vi "xiLIB - LoadPRMValue.vi"(6 "INI Refnum":T2, 7 "xiCam In":refnum<k24>, 8 "error in (no error)":errorcluster, 9 "key":string, 10 "section":string, 11 "PRM":T3) -> (0 "error out":errorcluster, 3 "Load_Result":T1, 4 "INI Refnum out":T2)   [LabVIEW 2015]
uses:
  <vilib>/Utility/config.llb/NI_LVConfig.lvlib
  <vilib>/Utility/config.llb/Read Key (Double).vi
  <vilib>/Utility/config.llb/Read Key (I32).vi
  Typedefs/xiLIB - PRM_Load_Result.ctl
  C:/GIT/Cameras3.x/Integrations/Labview/xiLib/xiLIB_32bit/xiLIB/xiCamLib/API/x86/xiApi.NET.dll
  xiLIB_32bit/xiLIB/xiCamLib/API/x86/xiApi.NET.dll
  <vilib>/Utility/config.llb/Config Data RefNum.ctl
  xiCam/PRM/PRM/PRM_v2.ctl
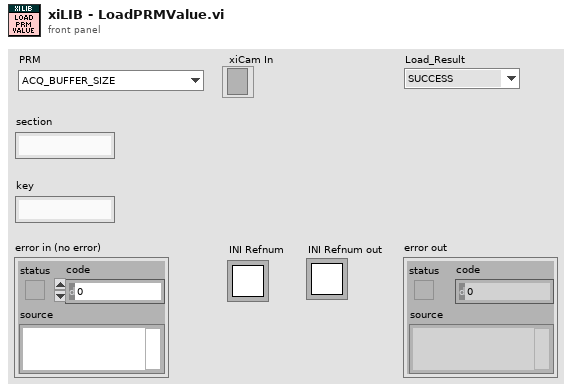
[diagram p1: front panel]
types:
  T1 = typedef "xiLIB - PRM_Load_Result.ctl" = enum16{"SUCCESS", "ERROR", "WARNING - Not Valid Parameter", "WARNING - Get Parameter"}
  T2 = typedef "NI_LVConfig.lvlib/Config Data RefNum.ctl" = refnum<k1>
  T3 = typedef "PRM_v2.ctl" = enum16{"ACQ_BUFFER_SIZE", "ACQ_FRAME_BURST_COUNT", "ACQ_TIMING_MODE", "ACQ_TRANSPORT_BUFFER_SIZE", "AE_MAX_LIMIT", "AEAG", "AEAG_LEVEL", "API_VERSION", "AG_MAX_LIMIT", "APPLY_CMS", "AUTO_BANDWIDTH_CALCULATION", "AUTO_WB", "AVAILABLE_BANDWIDTH", "AVAILABLE_BANDWIDTH_MAX", "AVAILABLE_BANDWIDTH_MIN", "BPC", "BUFFER_POLICY", "BUFFERS_QUEUE_SIZE", "CC_MATRIX_00", "CC_MATRIX_01", "CC_MATRIX_02", "CC_MATRIX_03", "CC_MATRIX_10", "CC_MATRIX_11", "CC_MATRIX_12", "CC_MATRIX_13", "CC_MATRIX_20", "CC_MATRIX_21", "CC_MATRIX_22", "CC_MATRIX_23", "CC_MATRIX_30", "CC_MATRIX_31", "CC_MATRIX_32", "CC_MATRIX_33", "CHIP_TEMP", "CMS", "COLOR_FILTER_ARRAY", "COOLING", "DEBOUNCE_EN", "DEBOUNCE_POL", "DEBOUNCE_T0", "DEBOUNCE_T1", "DEBUG_LEVEL", "DEFAULT_CC_MATRIX", "DEVICE_INSTANCE_PATH", "DEVICE_MODEL_ID", "DEVICE_NAME", "DEVICE_SN", "DEVICE_TYPE", "DEVICE_USER_ID", "DOWNSAMPLING", "DOWNSAMPLING_MAX", "DOWNSAMPLING_MIN", "DOWNSAMPLING_TYPE", "DRV_VERSION", "EXP_PRIORITY", "EXPOSURE", "EXPOSURE_DIRECT_UPDATE", "EXPOSURE_MAX", "EXPOSURE_MIN", "FFS_FILE_NAME", "FPGA1_VERSION", "FRAMERATE", "FRAMERATE_MAX", "FRAMERATE_MIN", "FREE_FFS_SIZE", "GAIN", "GAIN_DIRECT_UPDATE", "GAIN_MAX", "GAIN_MIN", "GAMMAC", "GAMMAY", "GPI_LEVEL", "GPI_MODE", "GPI_SELECTOR", "GPI_SELECTOR_MAX", "GPI_SELECTOR_MIN", "GPO_MODE", "GPO_SELECTOR", "GPO_SELECTOR_MAX", "GPO_SELECTOR_MIN", "HDR", "HDR_T1", "HDR_T2", "HEIGHT", "HEIGHT_MAX", "HEIGHT_MIN", "HOUSE_TEMP", "IMAGE_DATA_FORMAT", "IMAGE_IS_COLOR", "INPUT_CMS_PROFILE", "IS_COOLED", "IS_DEVICE_EXIST", "KNEEPOINT1", "KNEEPOINT2", "LED_MODE", "LED_SELECTOR", "LED_SELECTOR_MAX", "LED_SELECTOR_MIN", "LIMIT_BANDWIDTH", "LIMIT_BANDWIDTH_MAX", "LIMIT_BANDWIDTH_MIN", "LUT_EN", "LUT_INDEX", "LUT_INDEX_MAX", "LUT_INDEX_MIN", "LUT_VALUE", "LUT_VALUE_MAX", "LUT_VALUE_MIN", "MANUAL_WB", "MCU1_VERSION", "MCU2_VERSION", "OFFSET_X", "OFFSET_X_MAX", "OFFSET_X_MIN", "OFFSET_Y", "OFFSET_Y_MAX", "OFFSET_Y_MIN", "OUTPUT_CMS_PROFILE", "OUTPUT_DATA_BIT_DEPTH", "OUTPUT_DATA_PACKING", "READ_FILE_FFS", "RECENT_FRAME", "SENSOR_DATA_BIT_DEPTH", "SENSOR_MODE", "SENSOR_TAPS", "SHARPNESS", "SHUTTER_TYPE", "TARGET_TEMP", "TRG_DELAY", "TRG_SELECTOR", "TRG_SOFTWARE", "TRG_SOURCE", "USED_FFS_SIZE", "WB_KB", "WB_KG", "WB_KR", "WIDTH", "WIDTH_MAX", "WIDTH_MIN", "WRITE_FILE_FFS", "ACQ_BUFFER_SIZE_UNIT", "ACQ_TRANSPORT_BUFFER_COMMIT", "AEAG_ROI_HEIGHT", "AEAG_ROI_OFFSET_X", "AEAG_ROU_OFFSET_Y", "AEAG_ROI_WIDTH", "API_CONTEXT_LIST", "BINNING_HORIZONTAL", "BINNING_SELECTOR", "BINNING_VERTICAL", "COLUMN_FPN_CORRECTION", "COUNTER_SELECTOR", "COUNTER_VALUE", "DECIMATION_HORIZONTAL", "DECIMATION_SELECTOR", "DECIMATION_VERTICAL", "DEVICE_ID", "DEVICE_LOCATION_PATH", "DEVICE_MANIFEST", "DEVICE_RESET", "DEVICE_SENS_SN", "EXPOSURE_BURST_COUNT", "FFS_ACCESS_KEY", "GAIN_SELECTOR", "HW_REVISION", "IMAGE_BLACK_LEVEL", "IMAGE_DATA_BIT_DEPTH", "IMAGE_DATA_FORMAT_RGB32_ALPHA", "IMAGE_PAYLOAD_SIZE", "LENS_APERTURE_VALUE", "LENS_FEATURE", "LENS_FEATURE_SELECTOR", "LENS_FOCAL_LENGTH", "LENS_FOCUS_DISTANCE", "LENS_FOCUS_MOVE", "LENS_FOCUS_MOVEMENT_VALUE", "LENS_MODE", "OUTPUT_DATA_PACKING_TYPE", "SENSOR_CLOCK_FREQ_HZ", "SENSOR_CLOCK_FREQ_INDEX", "SENSOR_FEATURE_SELECTOR", "SENSOR_FEATURE_VALUE", "SENSOR_OUTPUT_CHANNEL_COUNT", "TRANSPORT_PIXEL_FORMAT", "TS_RST_MODE", "TS_RST_SOURCE"}
  T4 = typedef "xiLIB - PRM_Attribute.ctl" = cluster{"Type":T5, "Method":T6, "Desc.":string, "PRM":T3}
  T5 = typedef "xiLIB - PRM_Type.ctl" = enum16{"Int32", "Float", "String", "DOWNSAMPLING_TYPE", "IMAGE_DATA_FORMAT", "BUFFER_POLICY", "TRG_SOURCE", "GPI", "GPO", "ACQ_TIMING_MODE", "BINNING_PATTERN", "BINNING_SELECTOR", "CMS_MODE", "COUNTER_SELECTOR", "DEBUG_LEVEL", "DECIMATION_PATTERN", "DECIMATION_SELECTOR", "GAIN_SELECTOR_TYPE", "LED_MODE", "LENS_FEATURE_SELECTOR", "LENS_MODE", "OUTPUT_DATA_PACKING_TYPE", "SENSOR_FEATURE_SELECTOR", "SHUTTER_TYPE", "TRG_SELECTOR", "TS_RST_MODE", "TS_RST_SOURCE"}
  T6 = typedef "xiLIB - PRM_Function.ctl" = enum16{"Get / Set", "Get", "Set"}
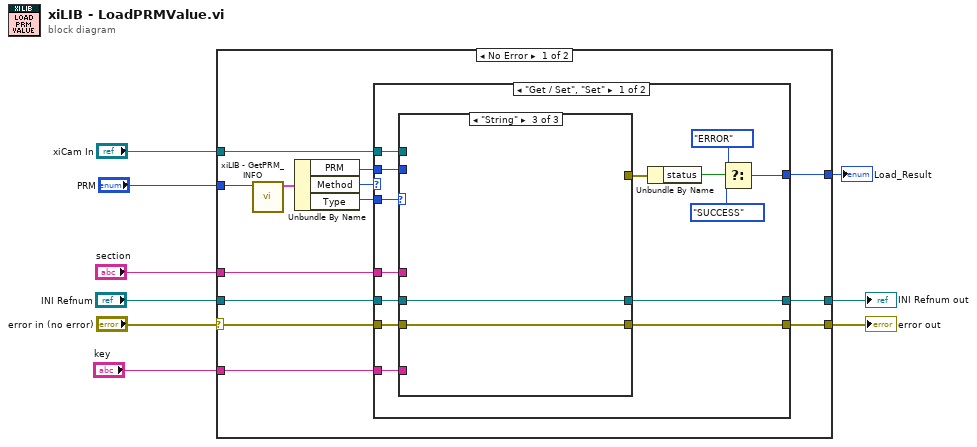
[diagram p0: block diagram]
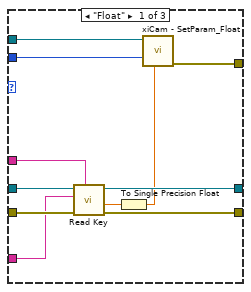
[diagram p2: hidden frame]
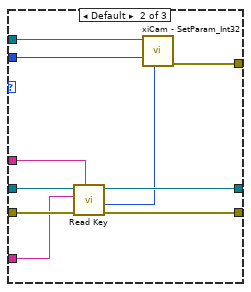
[diagram p3: hidden frame]
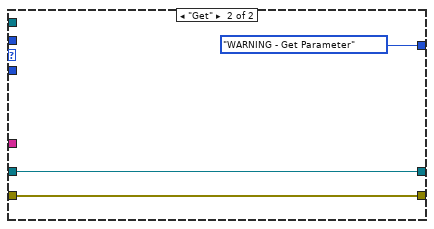
[diagram p4: hidden frame]
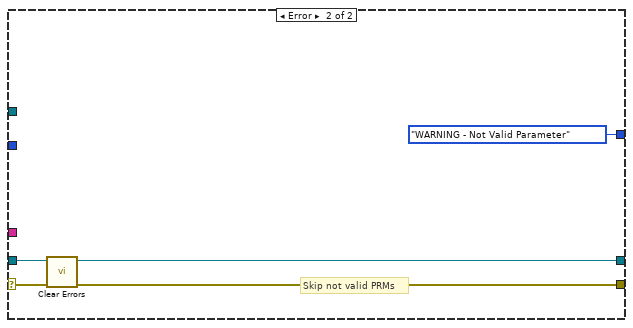
[diagram p5: hidden frame]
diagram:
  n1 = case shown="No Error" "error in (no error)" {
    selector: "error in (no error)" -> [w19 w66]
    tunnel: [w18 w64] -> w2
    tunnel: [w15 w65] -> w5
    tunnel: "xiCam In" -> [w17 _]
    tunnel: "PRM" -> [w14 _]
    tunnel: "INI Refnum" -> [w13 w64]
    tunnel: "key" -> [w12 _]
    tunnel: "section" -> [w11 _]
    tunnel: [w10 xiLIB_-_PRM_Load_Result."WARNING - Not Valid Parameter" ("Enum")] -> w1
    frame No Error {
      n2 = call "xiLIB - GetPRM_INFO.vi"("PRM"=w14) -> ("PRM_Attributes"=w22:T4)  [unwired: 10 in]
      n3 = Unbundle By Name(w22) -> ("PRM"=w16:T3, "Method"=w21:T6, "Type"=w20:T5)
      n4 = case shown="\"Get / Set\", \"Set\"" w21 {
        tunnel: w20 -> [w36 _]
        tunnel: w19 -> [w35 w62]
        tunnel: [w34 w61] -> w18
        tunnel: w17 -> [w33 _]
        tunnel: w16 -> [w32 _]
        tunnel: [w31 w62] -> w15
        tunnel: w13 -> [w29 w61]
        tunnel: w12 -> [w28 _]
        tunnel: w11 -> [w27 _]
        tunnel: [w23 xiLIB_-_PRM_Load_Result."WARNING - Get Parameter" ("Enum")] -> w10
        frame "Get / Set", "Set" {
          n5 = case shown="\"String\"" w36 {
            tunnel: w35 -> [w47 w57 w59]
            tunnel: [w46 w56 w58] -> w34
            tunnel: w33 -> [w44 w55 _]
            tunnel: w32 -> [w40 w51 _]
            tunnel: [w42 w54 _] -> w30
            tunnel: [w41 w53 w59] -> w31
            tunnel: w29 -> [w39 w50 w58]
            tunnel: w28 -> [w38 w49 _]
            tunnel: w27 -> [w37 w48 _]
            frame "Float" {
              n6 = call-poly <vilib>:"Read Key.vi"("section"=w37, "error in (no error)"=w47, "key"=w38, "refnum"=w39) -> ("error out"=w41:errorcluster, "value"=w45:dbl, "refnum out"=w46:T2)  [unwired: 4 in, 1 out]
              n7 = To Single Precision Float(number=w45) -> (single precision float=w43:sgl)
              n8 = call "xiCam - SetParam_Float.vi"("Float_Value"=w43, "PRM"=w40, "xiCam In"=w44) -> ("error out"=w42:errorcluster)  [unwired: 7 in, 1 out]
            }
            frame Default {
              n9 = call-poly <vilib>:"Read Key.vi"("section"=w48, "error in (no error)"=w57, "key"=w49, "refnum"=w50) -> ("error out"=w53:errorcluster, "value"=w52:i32, "refnum out"=w56:T2)  [unwired: 4 in, 1 out]
              n10 = call "xiCam - SetParam_Int32.vi"("Int32_Value"=w52, "PRM"=w51, "xiCam In"=w55) -> ("error out"=w54:errorcluster)  [unwired: 7 in, 1 out]
            }
            frame "String" {
            }
          }
          n11 = Unbundle By Name(w30) -> ("status"=w26:bool)
          n12 = Select(t=xiLIB_-_PRM_Load_Result."ERROR" ("Enum"), s=w26, f=xiLIB_-_PRM_Load_Result."SUCCESS" ("Enum")) -> (s? t:f=w23:T1)
        }
        frame "Get" {
        }
      }
    }
    frame Error {
      # "Skip not valid PRMs"
      n13 = call <vilib>:"Clear Errors.vi"("error in (no error)"=w66) -> ("error out"=w65:errorcluster)  [unwired: 5 in, 1 out]
    }
  }
  "error out" <- w5
  "INI Refnum out" <- w2
  "Load_Result" <- w1
